vi "setDC.vi"(0 "VISA Refnum in":refnum<visa-resource-name>, 1 "Output Response":T4=enum."Slow", 2 "Check For SCPI Errors? (T)":bool=TRUE, 3 "Turn Off Output If Voltage Limit?":bool=TRUE, 5 "Output State":T3, 7 "Analog Filter State":T3, 9 "Instrument Type":T5=enum."KE6221", 12 "Current Level (A)":T1 min=-0.105 max=0.105 format="%.4p", 13 "Voltage Limit (V)":T2 min=0.1 max=105.0 step=0.01 format="%.2p", 14 "Current Range In":T6={"Auto Range?"=TRUE, "Man / Selected\nRange"=enum."2nA"}) -> (4 "Interlock Tripped?":bool, 6 "Compliance?":bool, 15 "error out":errorcluster)   [LabVIEW 2023]
uses:
  <instrlib>/Keithley 622x LV 2009/Configure/Source/Typedefs/KE622x -- Current Range.ctl
  <instrlib>/Keithley 622x LV 2009/Configure/Source/Typedefs/KE622x -- Current Ranges.ctl
  Typedefs/KE622x -- On Off Control.ctl
  Kxx_Kxy_B_cs580_v3_LV20/Z/Labview Control Software/Keithley 622x LV 2009/Utility/Typedefs/KE622x -- Instrument Type.ctl
  Configure/Output/Typedefs/KE6221 -- Output Response.ctl
  Configure/Source/Typedefs/KE622x -- Voltage Limit.ctl
  <instrlib>/Keithley 622x LV 2009/Configure/Source/Typedefs/KE622x -- Current Level.ctl
  <instrlib>/Keithley 622x LV 2009/Keithley 622x.lvlib
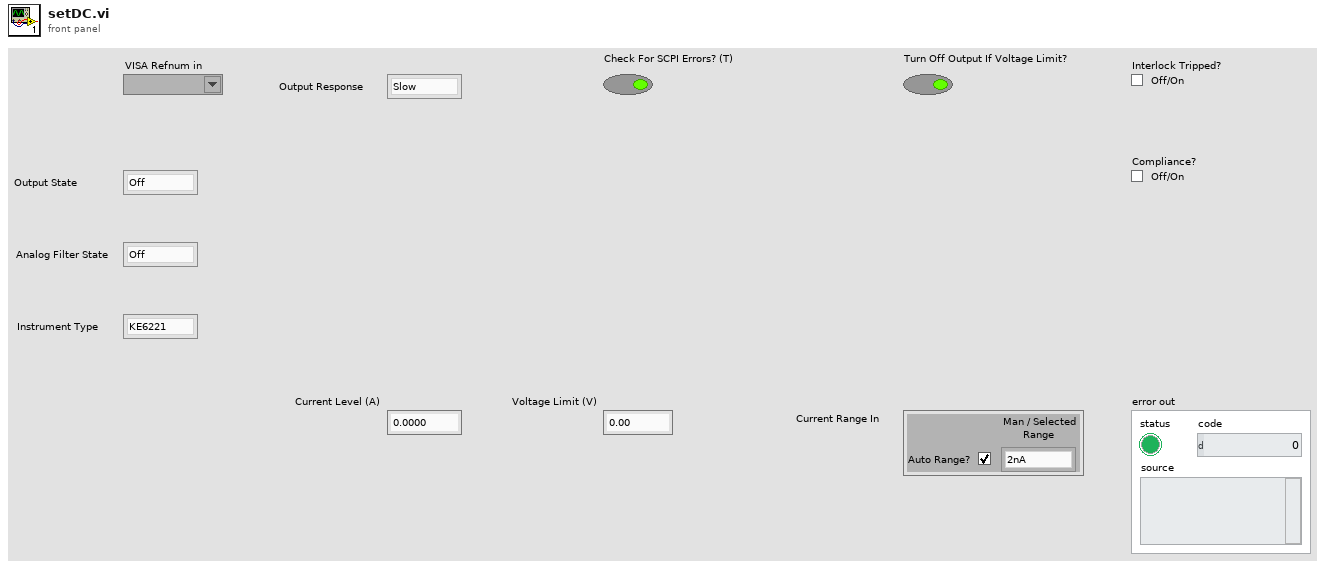
[diagram p1: front panel]
types:
  T1 = typedef "Keithley 622x.lvlib/KE622x -- Current Level.ctl" = dbl
  T2 = typedef "Keithley 622x.lvlib/KE622x -- Voltage Limit.ctl" = dbl
  T3 = typedef "Keithley 622x.lvlib/KE622x -- On Off Control.ctl" = enum16{"Off", "On"}
  T4 = typedef "Keithley 622x.lvlib/KE6221 -- Output Response.ctl" = enum16{"Fast", "Slow"}
  T5 = typedef "Keithley 622x.lvlib/KE622x -- Instrument Type.ctl" = enum16{"KE6220", "KE6221"}
  T6 = typedef "Keithley 622x.lvlib/KE622x -- Current Range.ctl" = cluster{"Auto Range?":bool, "Man / Selected\nRange":T7}
  T7 = typedef "Keithley 622x.lvlib/KE622x -- Current Ranges.ctl" = enum16{"2nA", "20nA", "200nA", "2uA", "20uA", "200uA", "2mA", "20mA", "100mA"}
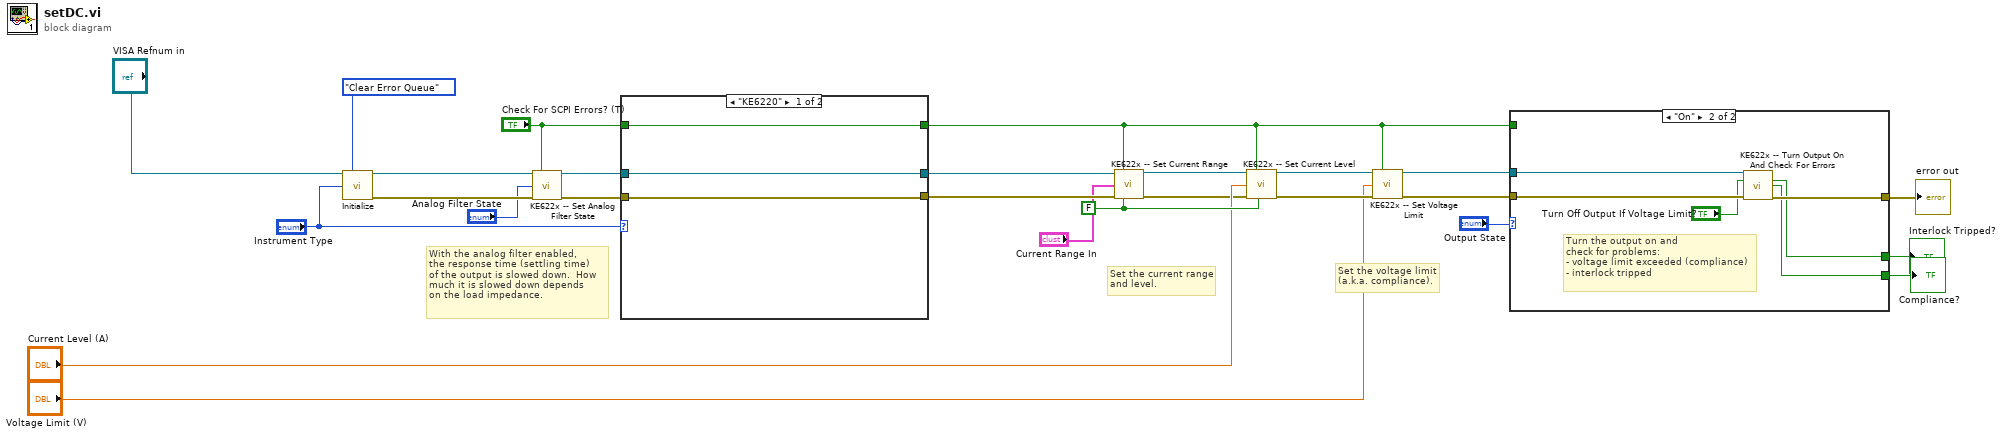
[diagram p0: block diagram]
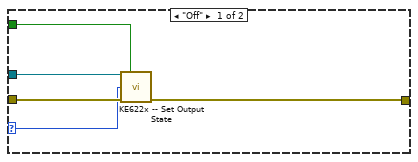
[diagram p2: hidden frame]
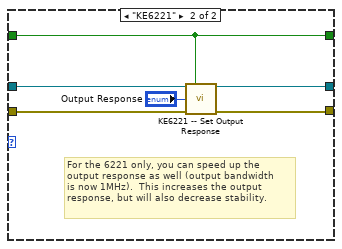
[diagram p3: hidden frame]
diagram:
  w16 = FALSE ("Read Back Set Values? (T)")
  # "Set the voltage limit\n(a.k.a. compliance)."
  # "Set the current range\nand level."
  # "With the analog filter enabled,\nthe response time (settling time)\nof the output is slowed down.  How\nmuch it is slowed down depends\non the load impedance."
  n1 = call "Initialize.vi"("VISA resource name"="VISA Refnum in", "Error Queue Option"=enum16{"Clear Error Queue", "Error Query"}."Clear Error Queue", "Instrument Type"="Instrument Type") -> ("VISA resource name out"=w5:refnum<visa-resource-name>, "error out"=w6:errorcluster)  [unwired: 11 in]
  n2 = call "KE622x -- Set Analog Filter State.vi"("Resource In"=w5, "Check For SCPI Errors? (T)"="Check For SCPI Errors? (T)", "Analog Filter State"="Analog Filter State", "error in (no error)"=w6) -> ("Resource Out (dupl)"=w7:refnum<visa-resource-name>, "error out"=w9:errorcluster)  [unwired: 10 in]
  n3 = case shown="\"KE6220\"" "Instrument Type" {
    tunnel: w7 -> [w28 w35]
    tunnel: w9 -> [w27 w33]
    tunnel: [w28 w32] -> w12
    tunnel: "Check For SCPI Errors? (T)" -> [w29 w31]
    tunnel: [w29 w31] -> w24
    tunnel: [w27 w30] -> w11
    frame "KE6220" {
    }
    frame "KE6221" {
      # "For the 6221 only, you can speed up the\noutput response as well (output bandwidth\nis now 1MHz).  This increases the output\nresponse, but will also decrease stability."
      n4 = call "KE6221 -- Set Output Response.vi"("Resource In"=w35, "Check For SCPI Errors? (T)"=w31, "KE6221 Output Response"="Output Response", "error in (no error)"=w33) -> ("Resource Out (dupl)"=w32:refnum<visa-resource-name>, "error out"=w30:errorcluster)  [unwired: 10 in]
    }
  }
  n5 = call <instrlib>:"KE622x -- Set Current Range.vi"("Resource In"=w12, "Check For SCPI Errors? (T)"=w24, "Current Range In"="Current Range In", "error in (no error)"=w11, "Read Back Set Values? (T)"=w16) -> ("Resource Out (dupl)"=w13:refnum<visa-resource-name>, "error out"=w14:errorcluster)  [unwired: 8 in, 1 out]
  n6 = call "KE622x -- Set Current Level.vi"("Resource In"=w13, "Check For SCPI Errors? (T)"=w24, "Current Level (A) In"="Current Level (A)", "error in (no error)"=w14, "Read Back Set Value? (T)"=w16) -> ("Resource Out (dupl)"=w18:refnum<visa-resource-name>, "error out"=w19:errorcluster)  [unwired: 8 in, 1 out]
  n7 = call "KE622x -- Set Voltage Limit.vi"("Resource In"=w18, "Check For SCPI Errors? (T)"=w24, "Voltage Limit (V)"="Voltage Limit (V)", "error in (no error)"=w19) -> ("Resource Out (dupl)"=w20:refnum<visa-resource-name>, "error out"=w21:errorcluster)  [unwired: 10 in]
  n8 = case shown="\"On\"" "Output State" {
    selector: "Output State" -> [w38 _]
    tunnel: w20 -> [w40 w46]
    tunnel: w21 -> [w39 w45]
    tunnel: [w36 w43] -> w22
    tunnel: w24 -> [w37 _]
    tunnel: [_ w42] -> w25
    tunnel: [_ w41] -> w26
    frame "Off" {
      n9 = call "KE622x -- Set Output State.vi"("Resource In"=w40, "Check For SCPI Errors? (T)"=w37, "Output State"=w38, "error in (no error)"=w39) -> ("error out"=w36:errorcluster)  [unwired: 10 in, 1 out]
    }
    frame "On" {
      # "Turn the output on and\ncheck for problems:\n- voltage limit exceeded (compliance)\n- interlock tripped"
      n10 = call "KE622x -- Turn Output On And Check For Errors.vi"("Resource In"=w46, "Turn Off Output If Compliance?"="Turn Off Output If Voltage Limit?", "error in (no error)"=w45) -> ("Interlock Tripped?"=w42:bool, "Compliance?"=w41:bool, "error out"=w43:errorcluster)  [unwired: 9 in, 1 out]
    }
  }
  "Compliance?" <- w26
  "Interlock Tripped?" <- w25
  "error out" <- w22
